vi "medicaoIXV.vi"() -> ()   [LabVIEW 2012]
uses:
  <vilib>/silver_ctls/ArrayMatrixCluster/Real Matrix NI_Silver.ctl
  <vilib>/Utility/file.llb/Write To Spreadsheet File (string).vi
  <vilib>/Utility/file.llb/Write To Spreadsheet File (DBL).vi
  <instrlib>/Agilent 6XXX Series/Agilent 6XXX Series.lvlib
  <vilib>/Analysis/NI_AALBase.lvlib
panel:
  out "tempSoma":dbl
  in  "x":dbl=10.0
  out "stopLoopMedicoes":bool caption="Parar Medição"
  out "desvio":dbl format="%0.2f"
  out "reset graph":bool=TRUE
  out "tabela":dbl[][](array[numeric])
  in  "Tab Control":enum32{"Entrada de dados", "Saída de dados"}(tab)
  in  "Irradiância":dbl caption="Irradiância(W/cm²)"
  in  "nCurvas":i64=1 caption="Nº de curvas" min=1
  in  "T.J":dbl caption="Tensão do joelho" step=0.1
  in  "p.a.j":dbl caption="Pontos antes do joelho"
  in  "nMedições":i16=1 caption="N° medições por ponto" min=1
  in  "area":dbl caption="Área da célula(cm²)"
  in  "Tipo":string caption="Tipo da célula"
  in  "Formato":u16(ring) items=[".txt", ".csv"]
  out "ON/OFF1":bool caption="ON/OFF"
  in  "p.d.j":dbl caption="Pontos depois do joelho"
  in  "T.M":dbl caption="Tensão máxima" step=0.1
  in  "Nome da célula":string
  in  "Local":path
  in  "Delay(ms)":dbl
  in  "Start":bool
  in  "temperatura":dbl caption="Temperatura da célula"
  out "tensaoFonte":dbl caption="Tensão da fonte (V)"
  out "Temp":dbl caption="Temperatura da célula (°C)"
  in  "stopProgram":bool caption="Parar Programa"
  out "Imp":dbl caption="Imp(A)"
  out "Vmp":dbl caption="Vmp(V)"
  out "Pmp":dbl caption="Pmp(W)"
  out "Icc (A)":dbl
  out "Vca (V)":dbl
  in  "Print Screen":bool caption="Screenshot da tela"
  out "IXV":cluster{"Y":dbl[], "Y":dbl[]}[](graph)
  out "vAtual":dbl caption="Tensao Atual (V)"
  out "iAtual":dbl caption="Corrente Atual (A)"
  out "Ponto Atual":i32
  out "tabela":T1 caption="TABELA DE DADOS\nTensão(Fonte)      Pontos             Tensao           Corrente"
  in  "stop":bool caption="Parar Medição"
  out "ON/OFF2":bool caption="ON/OFF"
  out "eficiencia":dbl caption="Eficiencia(%)"
  out "FF":dbl
  in  "CorrenteGraph":dbl
  in  "TensaoGraph":dbl
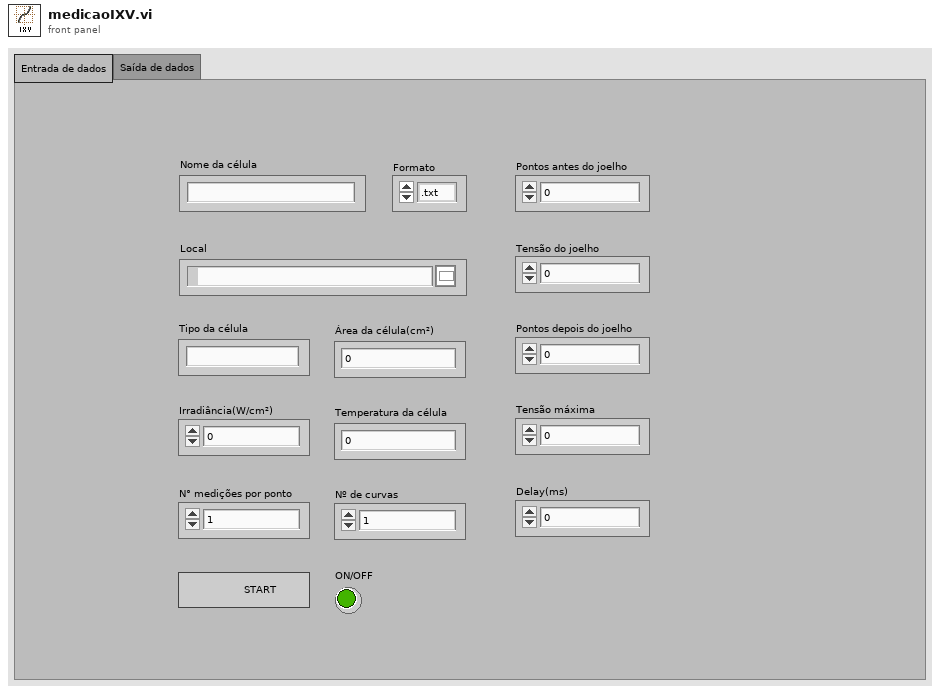
[diagram p1: front panel]
types:
  T1 = typedef "Real Matrix NI_Silver.ctl" = dbl[][]
  T2 = typedef "imagedata.ctl" = cluster{"image type":i32, "image depth":i32, "image":u8[], "mask":u8[], "colors":u32[], "Rectangle":cluster{"left":i16, "top":i16, "right":i16, "bottom":i16}}
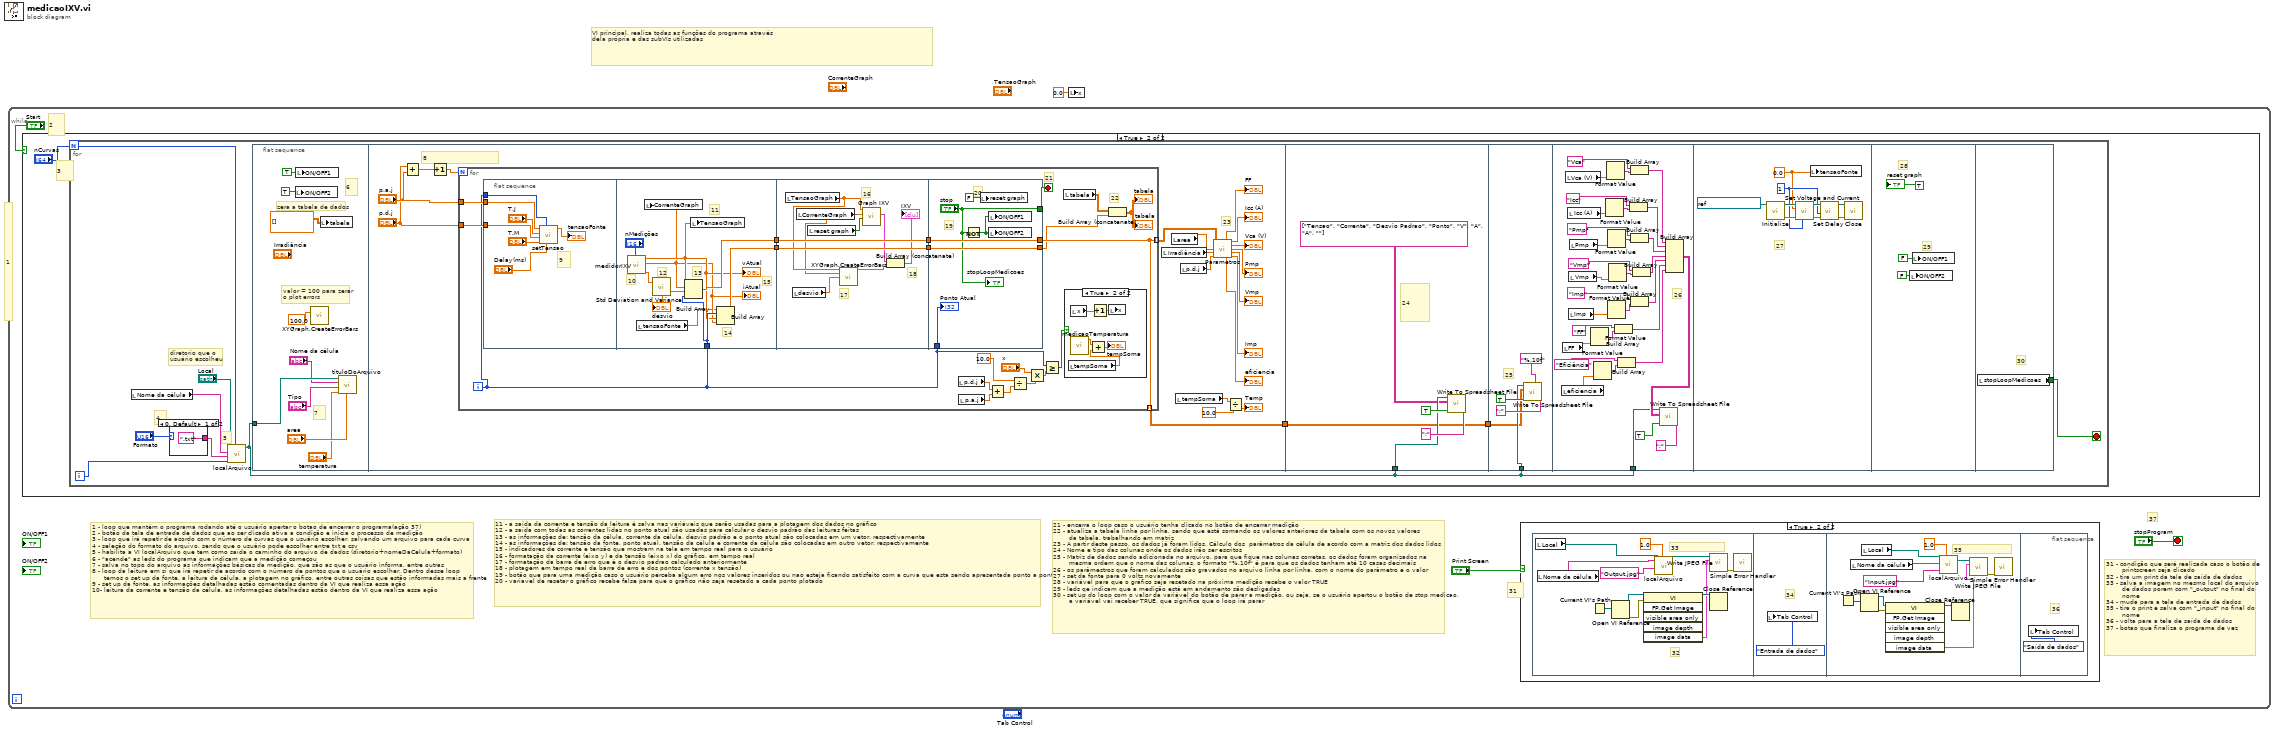
[diagram p0: block diagram]
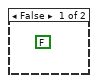
[diagram p3: hidden frame]
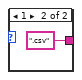
[diagram p4: hidden frame]
diagram:
  # "1"
  # "VI principal, realiza todas as funções do programa através \ndela própria e das subVIs utilizadas"
  n1 = while {
    stop <- "stopProgram" stop-if-true
    # "21 - encerra o loop caso o usuário tenha clicado no botão de encerrar medição\n22 - atualiza a tabela linha por linha, sendo que está somando os valores anteriores da tabela com os novos valores\n        da tabela, trabalhando em matriz\n23 - A partir deste passo, os dados já foram lidos. Cálculo dos  parâmetros da célula de acordo com a matriz dos dados lidos\n24 - Nome e tipo das colunas onde os dados irão ser escritos\n25 - Matriz de dados sendo adicionada no arquivo. para que fique nas colunas corretas, os dados foram organizados na \n        mesma ordem que o nome das colunas. o formato \"%.10f\" é para que os dados tenham até 10 casas decimais\n26 - os parâmestros que foram calculados são gravados no arquivo linha por linha, com o nome do parâmetro e o valor\n27 - set da fonte para 0 volts novamente \n28 - variável para que o gráfico seja resetado na próxima medição recebe o valor TRUE \n29 - leds qe indicam que a medição está em andamento são desligadas\n30 - set up do loop com o valor da variável do botão de parar a medição, ou seja, se o usuário apertou o botão de stop medicao,\n        a variável vai receber TRUE, que significa que o loop irá parar"
    # "11 - a saída da corrente e tensão da leitura é salva nas variáveis que serão usadas para a plotagem dos dados no gráfico\n12 - a saída com todas as correntes lidas no ponto atual são usadas para calcular o desvio padrão das leituras feitas\n13 - as informações de: tensão da célula, corrente da célula, desvio padrão e o ponto atual são colocadas em um vetor, respectivamente\n14 - as informações de: tensão da fonte, ponto atual, tensão da célula e corrente da célula são colocadas em outro vetor, respectivamente\n15 - indicadores de corrente e tensão que mostram na tela em tempo real para o usuário \n16 - formatação da corrente (eixo y) e da tensão (eixo x) do gráfico, em tempo real\n17 - formatação da barra de erro que é o desvio padrao calculado anteriormente\n18 - plotagem em tempo real da barra de erro e dos pontos (corrente x tensão)\n19 - botão que para uma medição caso o usuário perceba algum erro nos valores inseridos ou nao esteja ficando satisfeito com a curva que esta sendo apresentada ponto a ponto\n20 - variavel de resetar o gráfico recebe false para que o gráfico não seja resetado a cada ponto plotado"
    # "1 - loop que mantém o programa rodando até o usuário apertar o botao de encerrar o programa(ação 37)\n2 - botão da tela de entrada de dados que ao ser clicado ativa a condição e inicia o processo de medição\n3 - loop que irá repetir de acordo com o número de curvas que o usuário escolher, salvando um arquivo para cada curva \n4 - seleção do formato do arquivo, sendo que o usuário pode escolher entre txt e csv\n5 - habilita a VI localArquivo que tem como saída o caminho do arquivo de dados (diretorio+nomeDaCelula+formato) \n6 - \"acende\" as leds do programa que indicam que a medição começou\n7 - salva no topo do arquivo as informações básicas da medição, que são as que o usuário informa, entre outras\n8 - loop da leitura em si que irá repetir de acordo com o número de pontos que o usuário escolher. Dentro desse loop\n      temos o set up da fonte, a leitura da célula, a plotagem no gráfico, entre outras coisas que estão informadas mais a frente\n9 - set up da fonte, as informações detalhadas estão comentadas dentro da VI que realiza essa ação\n10- leitura da corrente e tensão da célula. as informações detalhadas estão dentro da VI que realiza essa ação"
    # "31 - condição que será realizada caso o botão de\n        printscreen seja clicado\n32 - tira um print da tela de saída de dados\n33 - salva a imagem no mesmo local do arquivo\n        de dados porem com \"_output\" no final do\n        nome\n34 - muda para a tela de entrada de dados\n35 - tira o print e salva com \"_input\" no final do\n        nome\n36 - volta para a tela de saída de dados \n37 - botao que finaliza o programa de vez"
    # "37"
    # "31"
    # "2"
    n2 = case shown="True" "Start" {
      frame False {
        (unwired) FALSE
      }
      frame True {
        # "3"
        n3 = for {
          N: "nCurvas" -> [w32]
          i -> [w31]
          stop <- w30 stop-if-true
          # "diretorio que o\nusuário escolheu"
          # "5"
          # "4"
          n4 = local read "Nome da célula"() -> (w35:string)
          n5 = case shown="0, Default" "Formato" {
            tunnel: [".txt" ".csv"] -> w34
            frame 0, Default {
            }
            frame 1 {
            }
          }
          n6 = call "localArquivo.vi"("quantidadeDeArquivos"=w32, "nAtualDoArquivo"=w31, "extensão"=w34, "Nome do arquivo"=w35, "Local"="Local") -> ("Path"=w33:path)  [unwired: 6 in]
          n7 = flat-sequence {
            tunnel: w33 -> [w50]
            tunnel: [w65] -> w39
            tunnel: w33 -> [w128]
            tunnel: [w127] -> w38
            tunnel: w39 -> [w127]
            tunnel: w33 -> [w132]
            tunnel: w38 -> [w131]
            tunnel: w33 -> [w144]
            tunnel: [w180] -> w30
            frame #0 {
              # "zera a tabela de dados"
              # "7"
              # "6"
              # "valor = 100 para zerar\no plot errors"
              n8 = local write "ON/OFF2"(TRUE ("ON/OFF2")) -> ()
              n9 = local write "ON/OFF1"(TRUE ("ON/OFF")) -> ()
              n10 = call "XYGraph.CreateErrorBars.vi"("yTemp"=100.0) -> ()  [unwired: 14 in, 1 out]
              n11 = local write "tabela"(dbl[][] [] ("array")) -> ()
              n12 = call "tituloDoArquivo.vi"("area"="area", "temperatura"="temperatura", "Tipo"="Tipo", "Nome da célula"="Nome da célula", "file path (dialog if empty)"=w50) -> ()  [unwired: 7 in]
            }
            frame #1 {
              # "23"
              # "8"
              n13 = Add(x="p.d.j", y="p.a.j") -> (x+y=w68:dbl)
              n14 = Increment(x=w68) -> (x+1=w69:dbl)
              n15 = for {
                N: w69 -> [_]
                tunnel: [w80] -> w58 mode=indexing
                tunnel: "p.a.j" -> [w82]
                tunnel: "p.d.j" -> [w81]
                tunnel: [w80] -> w65 mode=indexing
                i -> [w71]
                stop <- w85 stop-if-true
                # "22"
                # "21"
                n16 = flat-sequence {
                  tunnel: w71 -> [w101]
                  tunnel: w82 -> [w99]
                  tunnel: w81 -> [w98]
                  tunnel: w71 -> [w107]
                  tunnel: [w109] -> w89
                  tunnel: [w110] -> w88
                  tunnel: [w119] -> w84
                  tunnel: [w118] -> w83
                  tunnel: w88 -> [w118]
                  tunnel: w89 -> [w119]
                  tunnel: [w124] -> w79
                  tunnel: [w125] -> w80
                  tunnel: w84 -> [w125]
                  tunnel: w83 -> [w124]
                  tunnel: w71 -> [w123]
                  tunnel: ["stop"] -> w85
                  frame #0 {
                    # "9"
                    n17 = call "setTensao.vi"("delay(ms)"="Delay(ms)", "Ponto atual"=w101, "T.M"="T.M", "P.D.J"=w98, "T.J"="T.J", "P.A.J"=w99) -> ("output voltage"=→"tensaoFonte":dbl)  [unwired: 5 in]
                  }
                  frame #1 {
                    # "15"
                    # "14"
                    # "13"
                    # "11"
                    # "12"
                    # "10"
                    n18 = call "medidorIXV.vi"("nMedicoes"="nMedições") -> ("Tensao Atual"=w106:dbl, "Corrente Atual"=w105:dbl, "vetorCorrente"=w108:dbl[])  [unwired: 7 in]
                    "iAtual" <- w105
                    "vAtual" <- w106
                    n19 = local read "tensaoFonte"() -> (w102:dbl)
                    n20 = local write "CorrenteGraph"(w105) -> ()
                    n21 = call <vilib>:"Std Deviation and Variance.vi"("X"=w108) -> ("standard deviation"=w104:dbl)  [unwired: 1 in, 2 out]
                    "desvio" <- w104
                    n22 = Build Array(w106, w105, w104, w107) -> (w109:dbl[])
                    n23 = local write "TensaoGraph"(w106) -> ()
                    n24 = Build Array(w102, w107, w106, w105) -> (w110:dbl[])
                  }
                  frame #2 {
                    # "17"
                    # "18"
                    # "16"
                    n25 = local read "TensaoGraph"() -> (w113:dbl)
                    n26 = local read "desvio"() -> (w111:dbl)
                    n27 = local read "CorrenteGraph"() -> (w112:dbl)
                    n28 = local read "reset graph"() -> (w117:bool)
                    n29 = call "XYGraph.CreateErrorBars.vi"("xTemp"=w113, "yTemp"=w112, "errorTemp"=w111) -> ("error bar plot"=w114:cluster{dbl[], dbl[]})  [unwired: 12 in]
                    n30 = call "Graph IXV"("Reset"=w117, "Y Input"=w112, "X Input"=w113) -> ("XY Graph"=w116:cluster{"Y":dbl[], "Y":dbl[]}[])  [unwired: 2 in, 6 out]
                    n31 = Build Array (concatenate)(w116, w114) -> (→"IXV":cluster{"Y":dbl[], "Y":dbl[]}[])
                  }
                  frame #3 {
                    # "20"
                    # "19"
                    n32 = Not(x="stop") -> (.not. x?=w121:bool)
                    n33 = local write "reset graph"(FALSE) -> ()
                    n34 = local write "ON/OFF1"(w121) -> ()
                    n35 = local write "ON/OFF2"(w121) -> ()
                    "Ponto Atual" <- w123
                    "stopLoopMedicoes" <- "stop"
                  }
                }
                n36 = local read "p.d.j"() -> (w78:dbl)
                n37 = local read "p.a.j"() -> (w77:dbl)
                n38 = Add(x=w78, y=w77) -> (x+y=w76:dbl)
                n39 = Divide(x=10.0, y=w76) -> (x/y=w74:dbl)
                n40 = Multiply(x="x", y=w74) -> (x*y=w72:dbl)
                n41 = Greater Or Equal?(x=w71, y=w72) -> (x >= y?=w70:bool)
                n42 = local read "tabela"() -> (w87:dbl[][])
                n43 = case shown="True" w70 {
                  frame False {
                  }
                  frame True {
                    n44 = local read "tempSoma"() -> (w91:dbl)
                    n45 = local read "x"() -> (w93:dbl)
                    n46 = call "medicaoTemperatura.vi"() -> ("data"=w92:dbl)  [unwired: 11 in]
                    n47 = Add(x=w92, y=w91) -> (x+y=→"tempSoma":dbl)
                    n48 = Increment(x=w93) -> (x+1=w94:dbl)
                    n49 = local write "x"(w94) -> ()
                  }
                }
                n50 = Build Array (concatenate)(w87, w79) -> (→"tabela" →"tabela":dbl[][])
              }
              n51 = local read "Irradiância"() -> (w56:dbl)
              n52 = local read "area"() -> (w57:dbl)
              n53 = local read "tempSoma"() -> (w52:dbl)
              n54 = local read "p.d.j"() -> (w59:dbl)
              n55 = call "Parametros.vi"("VetorDeDados"=w58, "area"=w57, "irradiancia"=w56, "pontos"=w59) -> ("FF"=→"FF":dbl, "Icc"=→"Icc (A)":dbl, "Vca"=→"Vca (V)":dbl, "Pmp"=→"Pmp":dbl, "Vmp"=→"Vmp":dbl, "eficiencia"=→"eficiencia":dbl, "Imp"=→"Imp":dbl)  [unwired: 5 in]
              n56 = Divide(x=w52, y=10.0) -> (x/y=→"Temp":dbl)
            }
            frame #2 {
              # "24"
              n57 = call-poly <vilib>:"Write To Spreadsheet File.vi"("delimiter (\\t)"=";" ("delimiter (\\t)"), "append to file? (new file:F)"=TRUE, "2D data"=string[][] [["Tensao", "Corrente", "Desvio Padrao", "Ponto"], ["V", "A", "A", ""]], "file path (dialog if empty)"=w128) -> ()  [unwired: 4 in, 1 out]
            }
            frame #3 {
              # "25"
              n58 = call-poly <vilib>:"Write To Spreadsheet File.vi"("delimiter (\\t)"=";" ("delimiter (\\t)"), "format (%.3f)"="%.10f", "append to file? (new file:F)"=TRUE, "2D data"=w131, "file path (dialog if empty)"=w132) -> ()  [unwired: 3 in, 1 out]
            }
            frame #4 {
              # "26"
              n59 = local read "eficiencia"() -> (w138:dbl)
              n60 = local read "FF"() -> (w139:dbl)
              n61 = local read "Vca (V)"() -> (w146:dbl)
              n62 = local read "Icc (A)"() -> (w156:dbl)
              n63 = local read "Imp"() -> (w159:dbl)
              n64 = local read "Vmp"() -> (w158:dbl)
              n65 = local read "Pmp"() -> (w157:dbl)
              n66 = Format Value(value (0)=w139) -> (output string=w143:string)  [unwired: 2 in]
              n67 = Format Value(value (0)=w138) -> (output string=w142:string)  [unwired: 2 in]
              n68 = Format Value(value (0)=w156) -> (output string=w149:string)  [unwired: 2 in]
              n69 = Format Value(value (0)=w146) -> (output string=w147:string)  [unwired: 2 in]
              n70 = Format Value(value (0)=w157) -> (output string=w151:string)  [unwired: 2 in]
              n71 = Format Value(value (0)=w159) -> (output string=w155:string)  [unwired: 2 in]
              n72 = Format Value(value (0)=w158) -> (output string=w153:string)  [unwired: 2 in]
              n73 = Build Array("FF" ("string (\"\")"), w143) -> (w141:string[])
              n74 = Build Array("Eficiência" ("string (\"\")"), w142) -> (w140:string[])
              n75 = Build Array("Icc", w149) -> (w161:string[])
              n76 = Build Array("Vca", w147) -> (w160:string[])
              n77 = Build Array("Pmp", w151) -> (w162:string[])
              n78 = Build Array("Imp", w155) -> (w164:string[])
              n79 = Build Array("Vmp", w153) -> (w163:string[])
              n80 = Build Array(w160, w161, w162, w163, w164, w141, w140) -> (w165:string[][])
              n81 = call-poly <vilib>:"Write To Spreadsheet File.vi"("delimiter (\\t)"=";" ("delimiter (\\t)"), "append to file? (new file:F)"=TRUE, "2D data"=w165, "file path (dialog if empty)"=w144) -> ()  [unwired: 4 in, 1 out]
            }
            frame #5 {
              w168 = 0.0 ("voltage (0 V)")
              w171 = u8 1 ("channel (1)")
              # "27"
              n82 = call <instrlib>:"Initialize.vi"("VISA resource name"=refnum<visa-resource-name> "GPIB0::5::INSTR") -> ("error out"=w173:errorcluster, "VISA resource name out"=w172:refnum<visa-resource-name>)  [unwired: 9 in]
              n83 = call <instrlib>:"Set Voltage and Current.vi"("channel (1)"=w171, "error in (no error)"=w173, "voltage (0 V)"=w168, "VISA resource name"=w172) -> ("error out"=w174:errorcluster, "VISA resource name out"=w175:refnum<visa-resource-name>)  [unwired: 6 in]
              n84 = local write "tensaoFonte"(w168) -> ()
              n85 = call <instrlib>:"Set Delay.vi"("error in (no error)"=w174, "channel (1)"=w171, "VISA resource name"=w175) -> ("error out"=w169:errorcluster, "VISA resource name out"=w170:refnum<visa-resource-name>)  [unwired: 7 in]
              n86 = call <instrlib>:"Close.vi"("error in (no error)"=w169, "VISA resource name"=w170) -> ()  [unwired: 9 in, 1 out]
            }
            frame #6 {
              # "29"
              # "28"
              n87 = local write "ON/OFF2"(FALSE ("ON/OFF")) -> ()
              n88 = local write "ON/OFF1"(FALSE) -> ()
              "reset graph" <- TRUE
            }
            frame #7 {
              # "30"
              n89 = local read "stopLoopMedicoes"() -> (w180:bool)
            }
          }
        }
      }
    }
    n90 = case shown="True" "Print Screen" {
      frame False {
      }
      frame True {
        n91 = flat-sequence {
          frame #0 {
            # "33"
            # "32"
            n92 = local read "Local"() -> (w8:path)
            n93 = local read "Nome da célula"() -> (w6:string)
            n94 = Current VI's Path() -> (path=w13:path)
            n95 = Open VI Reference(vi path=w13) -> (vi reference=w14:refnum<vi>, error out=w15:errorcluster)  [unwired: 5 in]
            n96 = invoke class="VI" method="FP.Get Image"(reference=w14, error in=w15) -> (reference out=w12:refnum<vi>, "image data"=w11:T2)  [unwired: 4 in, 4 out]
            n97 = call "localArquivo.vi"("quantidadeDeArquivos"=1.0, "extensão"="Output.jpg", "Nome do arquivo"=w6, "Local"=w8) -> ("Path"=w5:path)  [unwired: 7 in]
            n98 = call <vilib>:"Write JPEG File.vi"("image data"=w11, "path to JPEG file"=w5) -> ("error out"=w10:errorcluster)  [unwired: 8 in, 1 out]
            n99 = Close Reference(reference=w12) -> ()  [unwired: 1 in, 1 out]
            n100 = call <vilib>:"Simple Error Handler.vi"("error in (no error)"=w10) -> ()  [unwired: 4 in, 5 out]
          }
          frame #1 {
            # "34"
            n101 = local write "Tab Control"(enum32{"Entrada de dados", "Saída de dados"}."Entrada de dados" ("Tab Control")) -> ()
          }
          frame #2 {
            # "35"
            n102 = Current VI's Path() -> (path=w26:path)
            n103 = local read "Nome da célula"() -> (w20:string)
            n104 = Open VI Reference(vi path=w26) -> (vi reference=w25:refnum<vi>, error out=w24:errorcluster)  [unwired: 5 in]
            n105 = local read "Local"() -> (w19:path)
            n106 = invoke class="VI" method="FP.Get Image"(reference=w25, error in=w24) -> (reference out=w27:refnum<vi>, "image data"=w22:T2)  [unwired: 4 in, 4 out]
            n107 = call "localArquivo.vi"("quantidadeDeArquivos"=1.0, "extensão"="Input.jpg", "Nome do arquivo"=w20, "Local"=w19) -> ("Path"=w18:path)  [unwired: 7 in]
            n108 = Close Reference(reference=w27) -> ()  [unwired: 1 in, 1 out]
            n109 = call <vilib>:"Write JPEG File.vi"("image data"=w22, "path to JPEG file"=w18) -> ("error out"=w23:errorcluster)  [unwired: 8 in, 1 out]
            n110 = call <vilib>:"Simple Error Handler.vi"("error in (no error)"=w23) -> ()  [unwired: 4 in, 5 out]
          }
          frame #3 {
            # "36"
            n111 = local write "Tab Control"(enum32{"Entrada de dados", "Saída de dados"}."Saída de dados" ("Tab Control")) -> ()
          }
        }
      }
    }
  }
  n112 = local write "x"(0.0 ("x")) -> ()
